vi "Ref_ROI_Translated_From_Ellipse_Center.vi"(10 "Ellipse Center":cluster{"Center X":dbl, "Center Y":dbl}, 11 "ROI Descriptor":T1 {"Contours"."Type" items=["No Selection", "Point", "Line", "Rectangle", "Oval", "Polygon", "Freehand Region", "Annulus", "Unused2", "Unused3", "Broken Line", "Freehand Line", "Rotated Rectangle"]}) -> (3 "Traslated ROI":T2)   [LabVIEW 2019, in "Algorithm.lvclass"]
uses:
  FrameworkOverrides/Algorithm.lvclass
types:
  T1 = typedef "ROI Descriptor" = cluster{"Global Rectangle":i32[], "Contours":cluster{"ID":enum32{"External", "Internal"}, "Type":u32, "Coordinates":i32[]}[]}
  T2 = cluster{"Left":dbl, "Top":dbl, "Right":dbl, "Bottom":dbl, "Angle":dbl}
  T3 = cluster{"ID":enum32{"External", "Internal"}, "Type":u32, "Coordinates":i32[]}[]
  T4 = cluster{"ID":enum32{"External", "Internal"}, "Type":u32, "Coordinates":i32[]}
  T5 = cluster{"Coordinates[0]":i32, "Coordinates[1]":i32, "Coordinates[2]":i32, "Coordinates[3]":i32, "Coordinates[4]":i32}
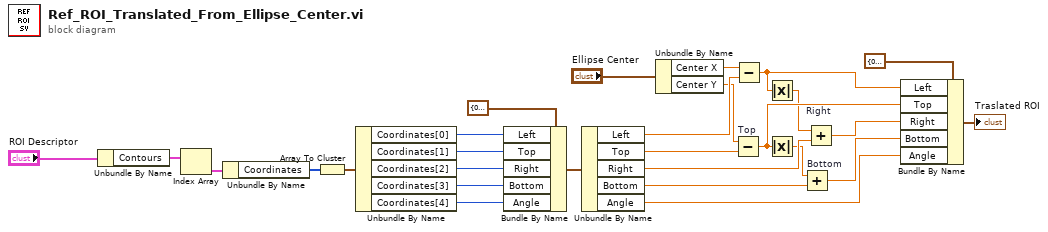
[diagram p0: block diagram]
diagram:
  n1 = Unbundle By Name("ROI Descriptor") -> ("Contours"=w28:T3)
  n2 = Index Array(array=w28) -> (element=w27:T4)  [unwired: 1 in]
  n3 = Unbundle By Name(w27) -> ("Coordinates"=w26:i32[])
  n4 = Array To Cluster(array=w26) -> (cluster=w25:T5)
  n5 = Unbundle By Name(w25) -> ("Coordinates[0]"=w23:i32, "Coordinates[1]"=w22:i32, "Coordinates[2]"=w21:i32, "Coordinates[3]"=w20:i32, "Coordinates[4]"=w19:i32)
  n6 = Bundle By Name(cluster=T2 {"Left"=0.0, "Top"=0.0, "Right"=0.0, "Bottom"=0.0, "Angle"=0.0} ("input cluster"), "Left"=w23, "Top"=w22, "Right"=w21, "Bottom"=w20, "Angle"=w19) -> (w6:T2)
  n7 = Unbundle By Name "Unbundle By Name"(w6) -> ("Left"=w14:dbl, "Top"=w15:dbl, "Right"=w16:dbl, "Bottom"=w17:dbl, "Angle"=w18:dbl)
  n8 = Unbundle By Name("Ellipse Center") -> ("Center X"=w4:dbl, "Center Y"=w5:dbl)
  n9 = Subtract "Top"(x=w5, y=w15) -> (x-y=w11:dbl)
  n10 = Subtract(x=w4, y=w14) -> (x-y=w10:dbl)
  n11 = Absolute Value(x=w10) -> (abs(x)=w7:dbl)
  n12 = Absolute Value(x=w11) -> (abs(x)=w8:dbl)
  n13 = Add "Bottom"(x=w8, y=w17) -> (x+y=w13:dbl)
  n14 = Add "Right"(x=w7, y=w16) -> (x+y=w12:dbl)
  n15 = Bundle By Name(cluster=T2 {"Left"=0.0, "Top"=0.0, "Right"=0.0, "Bottom"=0.0, "Angle"=0.0} ("input cluster"), "Left"=w10, "Top"=w11, "Right"=w12, "Bottom"=w13, "Angle"=w18) -> (→"Traslated ROI":T2)
